vi "State_Machine.vi"(8 "error in (no error)":errorcluster caption="entrée d'erreur (pas d'erreur)", 11 "Get_Voltage en entrée":refnum<class "Nodon_Set_Product_ID.lvclass">) -> (0 "error out":errorcluster caption="sortie d'erreur", 2 "Json_String":string, 3 "Get_Voltage en sortie":refnum<class "Nodon_Set_Product_ID.lvclass">)   [LabVIEW 2020, in "Library Test.lvlib" / "Nodon_Set_Product_ID.lvclass"]
uses:
  Nodon_Set_Product_ID.lvclass
  C:/Users/ngarcin/OneDrive - Altyor/Standard TB/Suite TB45/Class/Test/Test (Default)/Test (Default).lvclass
  C:/Users/ngarcin/OneDrive - Altyor/Standard TB/Suite TB45/Class/Test/Nodon_Send_Command_UART/Nodon_Send_Command_UART.lvclass
  Commun VI/TypeDef/Variable Printable.ctl
  JSON API/JSON Value/Set from JSON string.vi
  JSON API/JSON Value/JSON Value.lvclass
  Nodon_Send_Command_UART.lvclass
  JSON API/Variant JSON/Variant JSON.lvlib
  JSON API/Get Polymorphic/JSON GetSet.lvlib
  Commun VI/Library Commun.lvlib
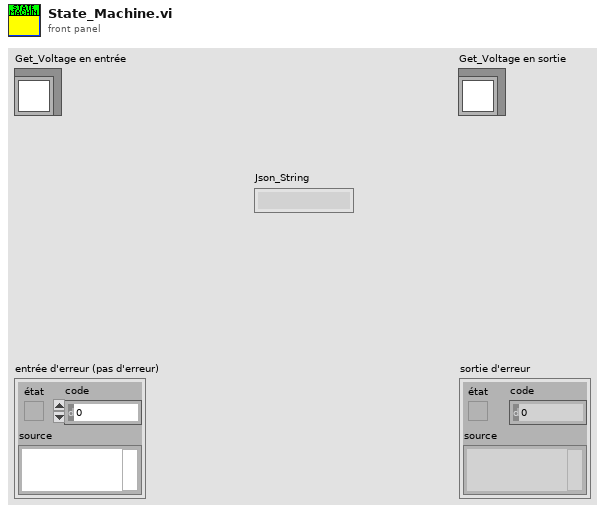
[diagram p1: front panel]
types:
  T1 = typedef "Variable Printable.ctl" = string
  T2 = enum16{"Get Variable", "Get All Variables", "Set Variable", "Delete Variable", "Delete All Variable"}
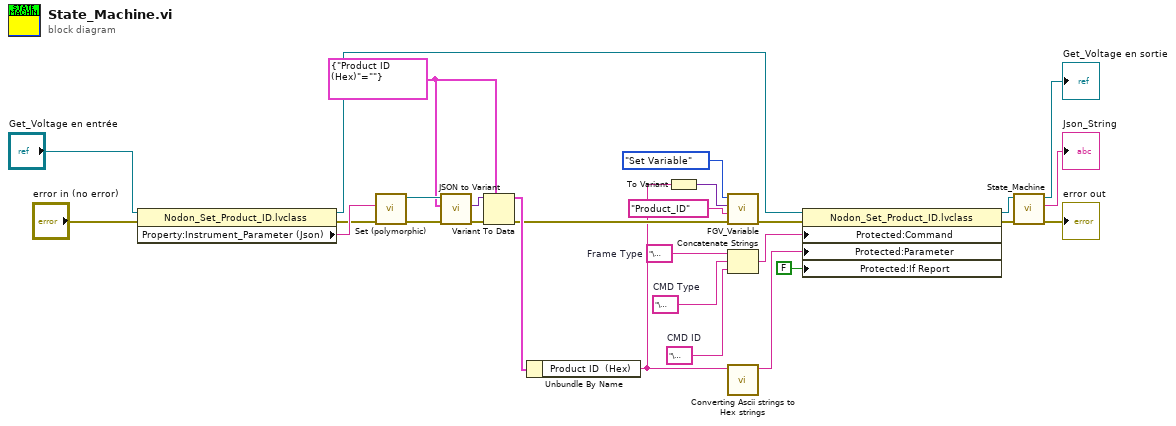
[diagram p0: block diagram]
diagram:
  w12 = cluster{"Product ID  (Hex)":string} {"Product ID  (Hex)"=""}
  w23 = "\u0000"  # Frame Type
  w22 = "\u0002"  # CMD ID
  w21 = "\u0003"  # CMD Type
  n1 = property class="Nodon_Set_Product_ID.lvclass"(reference="Get_Voltage en entrée", error in="error in (no error)") -> (reference out=w9:refnum<class "Nodon_Set_Product_ID.lvclass">, error out=w14:errorcluster, "Property:Instrument_Parameter (Json)"=w15:string)
  n2 = call-poly "Set (polymorphic).vi"("error in (no error)"=w14, "JSON stream"=w15) -> ("error out"=w17:errorcluster, "JSON Value out"=w19:refnum<class "JSON Value.lvclass">)  [unwired: 7 in, 1 out]
  n3 = call "JSON to Variant.vi"("error in (no error)"=w17, "Variant (Data Type)"=w12, "JSON Value"=w19) -> ("error out"=w18:errorcluster, "Variant out"=w16:variant)  [unwired: 7 in]
  n4 = Variant To Data(error in=w18, type=w12, Variant=w16) -> (data=w11:cluster{"Product ID  (Hex)":string}, error out=w4:errorcluster)
  n5 = Unbundle By Name(w11) -> ("Product ID  (Hex)"=w3:string)
  n6 = To Variant(anything=w3) -> (Variant=w2:variant)
  n7 = call "FGV_Variable.vi"("error in (no error)"=w4, "Variable"=T1 "Product_ID", "Data In"=w2, "Function"=T2."Set Variable") -> ("error out"=w1:errorcluster)  [unwired: 5 in, 2 out]
  n8 = Concatenate Strings(w23, w21, w22) -> (w20:string)
  n9 = call "Converting Ascii strings to Hex strings.vi"("result string"=w3) -> ("Chaîne"=w7:string)  [unwired: 10 in]
  n10 = property class="Nodon_Set_Product_ID.lvclass"(reference=w9, error in=w1, "Protected:Command"=w20, "Protected:Parameter"=w7, "Protected:If Report"=FALSE ("If Report")) -> (reference out=w25:refnum<class "Nodon_Set_Product_ID.lvclass">, error out=w24:errorcluster)
  n11 = call-parent "State_Machine.vi"("error in (no error)"=w24, "Send_Frame en entrée"=w25) -> ("error out"=→"error out":errorcluster, "Json_String"=→"Json_String":string, "Send_Frame en sortie"=→"Get_Voltage en sortie":refnum<class "Nodon_Set_Product_ID.lvclass">)  [unwired: 7 in]
